vi "set Stufentabelle.vi"(6 "Index in":T1, 8 "Fehler (Eingang, kein Fehler)":errorcluster, 9 "Komponente in":T3, 10 "Table Index":i32, 11 "GD in":T4) -> (0 "Fehler (Ausgang)":errorcluster, 1 "Komponente out":T3, 2 "EGAK":T2[](array[typedef]), 3 "Stufen Tabellen out":string[][](array[string]))   [LabVIEW 2020, in "Linearisierung v2.lvlib" / "SpanEinstellungen.lvlib"]
uses:
  SpanEinstellungen.lvlib
  Visualisierungs Elemente/Auswahlfeld.ctl
  Seiten/System Einstellungen V2/Traegergas.ctl
  Aktion Lin Daten aufarbeiten.ctl
  Aktion FGV SPAN Stufentabellen.ctl
  Linearisierung v2.lvlib
  Seiten/System Einstellungen V2/System Einstellungen V2.lvlib
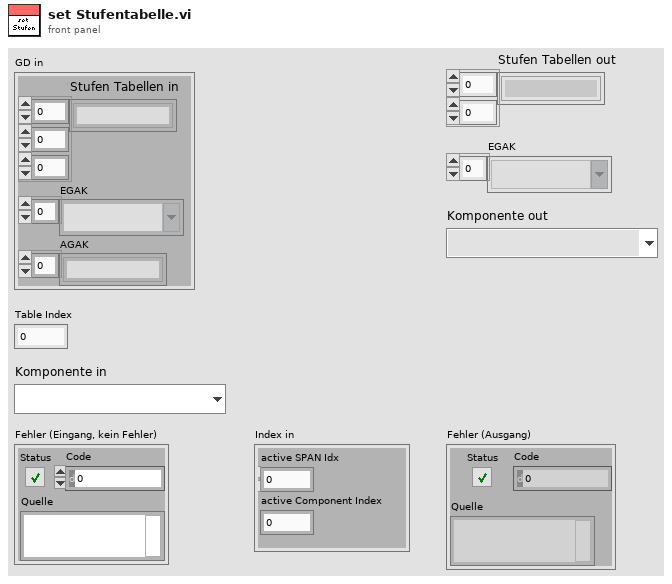
[diagram p1: front panel]
types:
  T1 = cluster{"active SPAN Idx":i32, "active Component Index":i32}
  T2 = typedef "System Einstellungen V2.lvlib/Traegergas.ctl" = string
  T3 = typedef "Auswahlfeld.ctl" = u16
  T4 = cluster{"Stufen Tabellen in":string[][][], "EGAK":T2[], "AGAK":string[]}
  T5 = typedef "Linearisierung v2.lvlib/SpanEinstellungen.lvlib/Aktion FGV SPAN Stufentabellen.ctl" = enum16{"lesen", "schreiben", "init"}
  T6 = typedef "Linearisierung v2.lvlib/Aktion Lin Daten aufarbeiten.ctl" = enum16{"lesen", "Protkolldaten", "speichern", "laden", "EPA auswerten", "Tabelle schreiben", "Lin auswerten", "Tab init", "Stufentabelle", "EPA aktiviert", "Nachbehandlung laden", "Tabelle löschen", "Istwerte löschen", "Zeile löschen", "Zeile einfügen", "LIN aktiviert", "LIN/EPA aktiv laden", "EGAK Tab", "LIN übernehmen", "Tab init ohne Stufen"}
  T7 = cluster{"active SPAN Idx":i32, "active Component Index":i32, "Stufen Tabellen in":string[][], "EGAK":T2[]}
  T8 = typedef "Linearisierung v2.lvlib/Gasteiler.lvlib/Stufen Tabelle.ctl" = string[][]
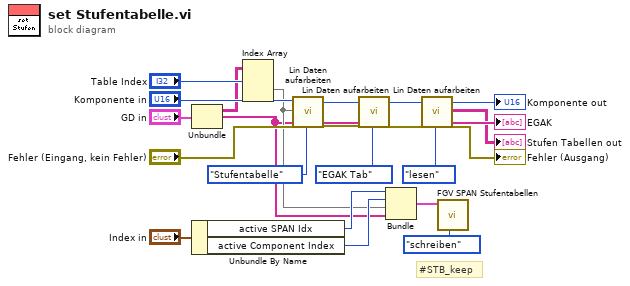
[diagram p0: block diagram]
diagram:
  # "#STB_keep"
  n1 = Unbundle("GD in") -> ("Stufen Tabellen in"=w16:string[][][], "EGAK"=w1:T2[])  [unwired: 1 out]
  n2 = Unbundle By Name("Index in") -> ("active SPAN Idx"=w6:i32, "active Component Index"=w5:i32)
  n3 = Index Array(array=w16, index (dim 0)="Table Index") -> (element=w2:string[][])  [unwired: 2 in]
  n4 = call "Lin Daten aufarbeiten.vi"("Index (Seite)"="Komponente in", "Stufen Tabelle"=w2, "error in (no error)"="Fehler (Eingang, kein Fehler)", "Aktionen"=Aktion_Lin_Daten_aufarbeiten."Stufentabelle") -> ("Index (Seite) out"=w18:i32, "error out"=w21:errorcluster)  [unwired: 13 in, 9 out]
  n5 = call "Lin Daten aufarbeiten.vi"("Index (Seite)"=w18, "EGAK"=w1, "error in (no error)"=w21, "Aktionen"=Aktion_Lin_Daten_aufarbeiten."EGAK Tab") -> ("Index (Seite) out"=w14:i32, "error out"=w10:errorcluster)  [unwired: 13 in, 9 out]
  n6 = Bundle("active SPAN Idx"=w6, "active Component Index"=w5, "Stufen Tabellen in"=w2, "EGAK"=w1) -> (w3:T7)  [unwired: 1 in]
  n7 = call "Lin Daten aufarbeiten.vi"("Index (Seite)"=w14, "error in (no error)"=w10, "Aktionen"=Aktion_Lin_Daten_aufarbeiten."lesen") -> ("Index (Seite) out"=→"Komponente out":i32, "Stufen Tabelle"=→"Stufen Tabellen out":T8, "EKAG"=→"EGAK":string[], "error out"=→"Fehler (Ausgang)":errorcluster)  [unwired: 14 in, 7 out]
  n8 = call "FGV SPAN Stufentabellen.vi"("Aktion"=Aktion_FGV_SPAN_Stufentabellen."schreiben", "In Cluster"=w3) -> ()  [unwired: 5 in, 4 out]
